vi "PH_4_Pos_Selector.Picture Default.vi"(1 "Current Position":T1 items=["unknown", "Position I", "Position II", "Position III", "Position IV", "moving"]) -> (0 "Default Array":picture[](array[picture]))   [LabVIEW 2014, in "PH_4_Pos_Selector.lvlib"]
uses:
  PH_4_Pos_Selector.lvlib
  PH_4_Pos_Selector.Position Selector.ctl
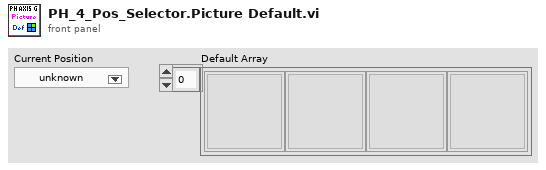
[diagram p1: front panel]
types:
  T1 = typedef "PH_4_Pos_Selector.lvlib/PH_4_Pos_Selector.Position Selector.ctl" = u16
  T2 = cluster{"left":i16, "top":i16, "right":i16, "bottom":i16}
  T3 = enum16{"User-specified Font", "Application Font", "System Font", "Dialog Font"}
  T4 = cluster{"Font Name:":string, "Size":i16, "Strikeout?":bool, "Italic?":bool, "Underline?":bool, "Outline?":bool, "Shadow?":bool, "Bold?":bool}
  T5 = cluster{"horizontal":enum16{"left", "center", "right"}, "vertical":enum16{"top", "center", "bottom"}}
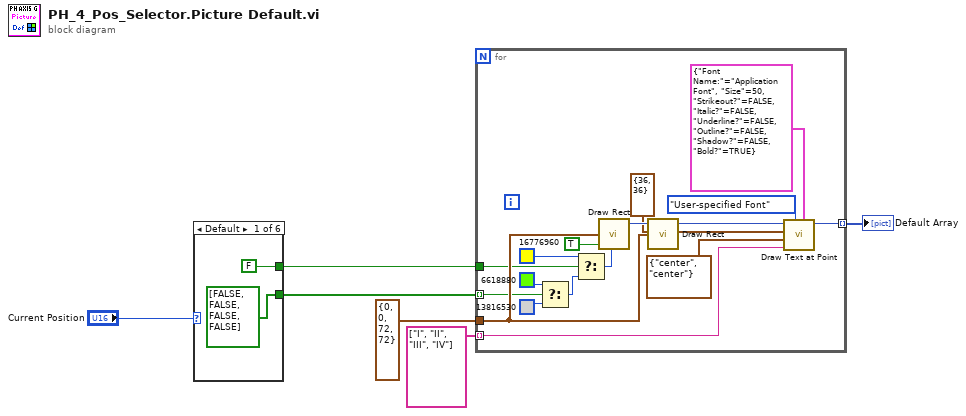
[diagram p0: block diagram]
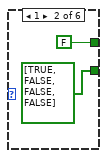
[diagram p2: hidden frame]
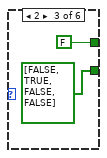
[diagram p3: hidden frame]
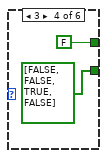
[diagram p4: hidden frame]
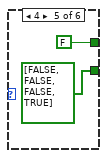
[diagram p5: hidden frame]
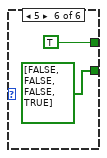
[diagram p6: hidden frame]
diagram:
  n1 = case shown="Default" "Current Position" {
    tunnel: [bool[] [FALSE, FALSE, FALSE, FALSE] bool[] [TRUE, FALSE, FALSE, FALSE] bool[] [FALSE, TRUE, FALSE, FALSE] bool[] [FALSE, FALSE, TRUE, FALSE] bool[] [FALSE, FALSE, FALSE, TRUE] bool[] [FALSE, FALSE, FALSE, TRUE]] -> w5
    tunnel: [FALSE FALSE FALSE FALSE FALSE TRUE] -> w4
    frame Default {
    }
    frame 1 {
    }
    frame 2 {
    }
    frame 3 {
    }
    frame 4 {
    }
    frame 5 {
    }
  }
  n2 = for {
    tunnel: T2 {"left"=0, "top"=0, "right"=72, "bottom"=72} ("rect") -> [w34]
    tunnel: w5 -> [w33] mode=indexing
    tunnel: w4 -> [w28]
    tunnel: [w20] -> w2 mode=indexing
    tunnel: string[] ["I", "II", "III", "IV"] -> [w21] mode=indexing
    n3 = Select(t=u32 6618880, s=w33, f=u32 13816530) -> (s? t:f=w26:u32)
    n4 = Select(t=u32 16776960, s=w28, f=w26) -> (s? t:f=w25:u32)
    n5 = call <vilib>:"Draw Rect.vi"("rect"=w34, "fill?(F)"=TRUE, "color(black)"=w25) -> ("new picture"=w35:picture)  [unwired: 6 in]
    n6 = call <vilib>:"Draw Rect.vi"("picture"=w35, "rect"=w34) -> ("new picture"=w29:picture)  [unwired: 7 in]
    n7 = call <vilib>:"Draw Text at Point.vi"("[user-specified font]"=T4 {"Font Name:"="Application Font", "Size"=50, "Strikeout?"=FALSE, "Italic?"=FALSE, "Underline?"=FALSE, "Outline?"=FALSE, "Shadow?"=FALSE, "Bold?"=TRUE}, "desired font(Application)"=T3."User-specified Font", "text"=w21, "alignment(left, top)"=T5 {"horizontal"=enum."center", "vertical"=enum."center"}, "origin"=cluster{"x":i16, "y":i16} {"x"=36, "y"=36}, "picture"=w29) -> ("new picture"=w20:picture)  [unwired: 4 in, 1 out]
  }
  "Default Array" <- w2
